vi "sourcemeter and electrometer.vi"() -> ()   [LabVIEW 2018]
panel:
  out "Waveform Chart":dbl(graph)
  out "Numeric":dbl format="%#_13g"
  in  "stop":bool
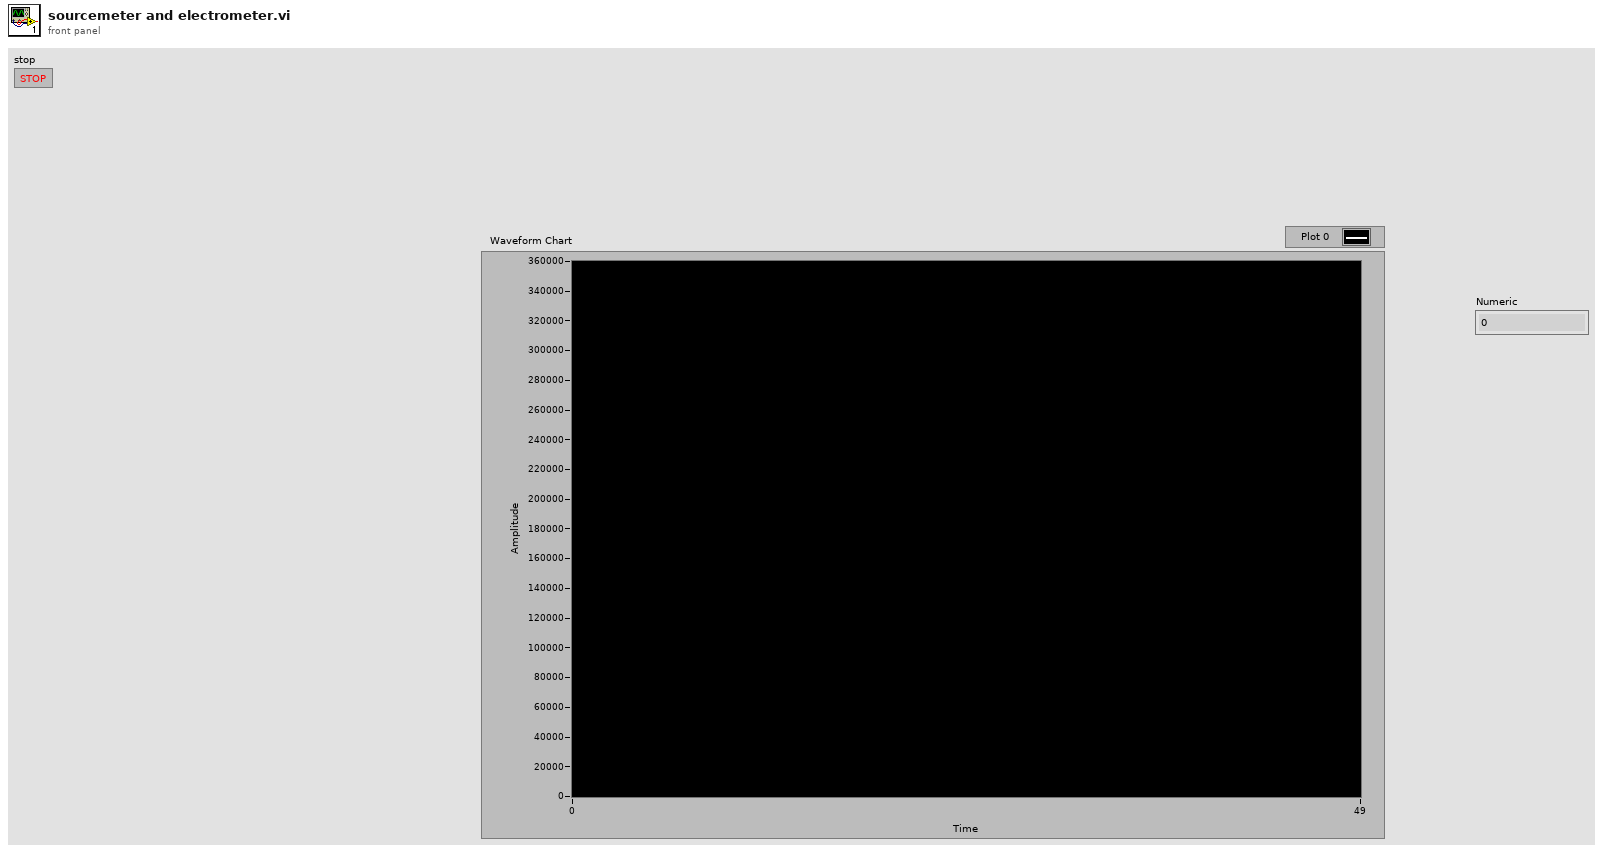
[diagram p1: front panel]
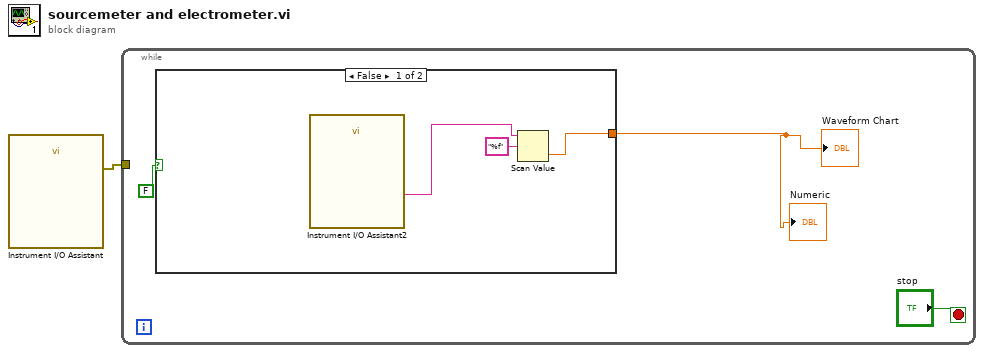
[diagram p0: block diagram]
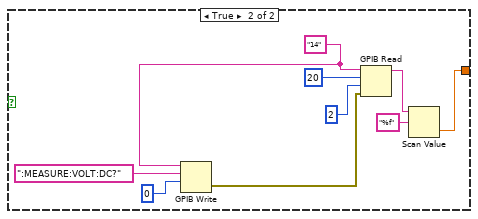
[diagram p2: hidden frame]
diagram:
  n1 = call "Instrument I/O Assistant"() -> ("error out"=w1:errorcluster)  [unwired: 24 in, 3 out]
  n2 = while {
    tunnel: w1 -> [_]
    stop <- "stop" stop-if-true
    n3 = case shown="False" FALSE ("Boolean") {
      tunnel: [w5 w9] -> w2
      frame False {
        n4 = call "Instrument I/O Assistant2"() -> ("token"=w6:string)  [unwired: 24 in, 3 out]
        n5 = Scan Value(string=w6, format string="%f") -> (value=w5:dbl)  [unwired: 1 in, 1 out]
      }
      frame True {
        w14 = "14" ("address string")
        n6 = GPIB Write(0:w14, 1:":MEASURE:VOLT:DC?" ("write buffer"), 2:i16 0 ("mode (0)")) -> (6:w13:errorcluster)  [unwired: 2 in, 1 out]
        n7 = GPIB Read(0:w14, 1:20 ("byte count"), 2:i16 2 ("mode (0)"), 3:w13) -> (5:w10:string)  [unwired: 1 in, 2 out]
        n8 = Scan Value(string=w10, format string="%f") -> (value=w9:dbl)  [unwired: 1 in, 1 out]
      }
    }
    "Numeric" <- w2
    "Waveform Chart" <- w2
  }
